vi "RT_Listener Loop.vi"(8 "error in":errorcluster, 11 "Main Data":T1) -> ()   [LabVIEW 2018]
uses:
  Data Def/RT_Main Data.ctl
  Data Def/RT_FPGA VI Reference.ctl
  Data Def/RT_Request Data.ctl
  Com/WebSockets/Data Def/WebSocket Manerger Method.ctl
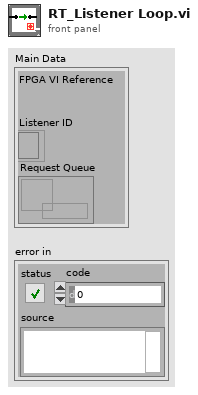
[diagram p1: front panel]
types:
  T1 = typedef "RT_Main Data.ctl" = cluster{"FPGA VI Reference":T2, "Listener ID":refnum<k5>, "Request Queue":refnum<queue>}
  T2 = typedef "RT_FPGA VI Reference.ctl" = refnum<k20>
  T3 = typedef "WebSocket Manerger Method.ctl" = enum16{"Initialize", "Add Connection", "Get Connections", "Close Connection", "Close All"}
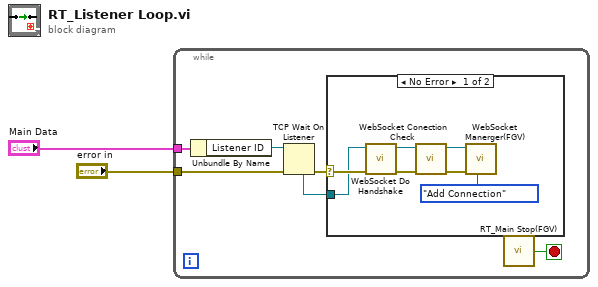
[diagram p0: block diagram]
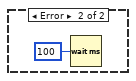
[diagram p2: hidden frame]
diagram:
  n1 = while {
    tunnel: "error in" -> [w5]
    tunnel: "Main Data" -> [w4]
    stop <- w3 stop-if-true
    n2 = Unbundle By Name(w4) -> ("Listener ID"=w8:refnum<k5>)
    n3 = TCP Wait On Listener(8:w5, 11:w8) -> (0:w7:errorcluster, 4:w6:refnum<k5>)  [unwired: 2 in, 3 out]
    n4 = case shown="No Error" w7 {
      selector: w7 -> [w15 _]
      tunnel: w6 -> [w14 _]
      frame No Error {
        n5 = call "WebSocket Do Handshake.vi"("error in (no error)"=w15, "WebSocket Connection in"=w14) -> ("error out"=w13:errorcluster, "WebSocket Connection out"=w12:refnum<k5>)  [unwired: 6 in, 2 out]
        n6 = call "WebSocket Conection Check.vi"("error in"=w13, "Connection In"=w12) -> ("error out"=w11:errorcluster, "Connection Out"=w10:refnum<k5>)  [unwired: 8 in]
        n7 = call "WebSocket Manerger(FGV).vi"("WebSocket Manerger Method"=WebSocket_Manerger_Method."Add Connection", "error in"=w11, "connection In"=w10) -> ()  [unwired: 7 in, 2 out]
      }
      frame Error {
        n8 = Wait (ms)(milliseconds to wait=u32 100) -> ()  [unwired: 1 out]
      }
    }
    n9 = call "RT_Main Stop(FGV).vi"() -> ("Stop Out"=w3:bool)  [unwired: 4 in]
  }
